vi "TellSelf.vi"(10 "Message":T1 {"MessageMetadata"."AbsoluteTime" format="%<%x %.3X>T"}, 11 "Actor":refnum<class "Actor.lvclass">) -> (0 "Error":errorcluster, 3 "Actor":refnum<class "Actor.lvclass">)   [LabVIEW 2020, in "_Template.lvlib" / "Templates.lvlib" / "{{Name}}Message.lvlib"]
uses:
  {{Name}}Message.lvlib
  {{Name}}Message/{{Name}}Message.lvclass
  C:/jettl-harness/repos/jettl/src/jettl Tools/_Template/Templates/{{Name}}Message/{{Name}}Message/{{Name}}Message.lvclass
  C:/jettl-harness/repos/jettl/src/jettl/jettl/Message/Message.lvclass
  jettl/jettl/jettl.lvlib
  jettl/jettl/Actor/Actor.lvclass
  jettl/jettl/ActorRelation.ctl
  jettl/jettl/ActorLifetime.ctl
  jettl/jettl/MessageMetadata.ctl
  Message.ctl
panel:
  # "This front panel should not be manipulated."
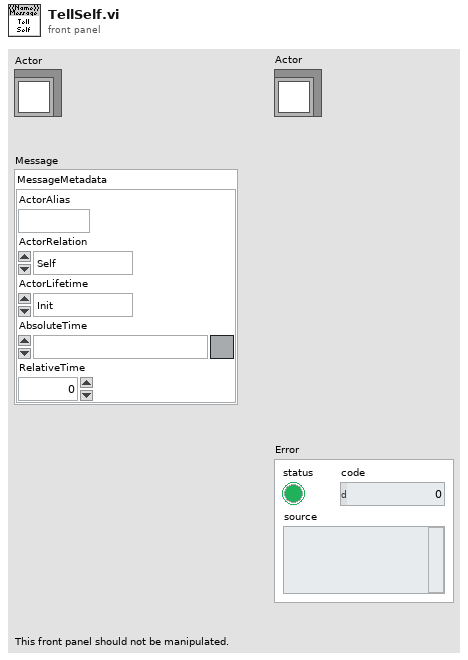
[diagram p1: front panel]
types:
  T1 = typedef "_Template.lvlib/Templates.lvlib/{{Name}}Message.lvlib/Message.ctl" = cluster{"MessageMetadata":T2}
  T2 = typedef "jettl.lvlib/MessageMetadata.ctl" = cluster{"ActorAlias":string, "ActorRelation":T3, "ActorLifetime":T4, "AbsoluteTime":timestamp, "RelativeTime":dbl}
  T3 = typedef "jettl.lvlib/ActorRelation.ctl" = enum16{"Self", "Actor"}
  T4 = typedef "jettl.lvlib/ActorLifetime.ctl" = enum16{"Init", "Spawn", "Setup", "Teardown Before Running", "Running", "Stop Called", "Stopping With Children", "Stopping Without Children", "Teardown After Running", "Stopped"}
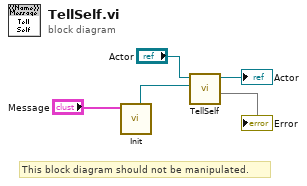
[diagram p0: block diagram]
diagram:
  # "This block diagram should not be manipulated."
  n1 = call "Init.vi"("Message"="Message") -> ("{{Name}}Message"=w5:refnum<class "{{Name}}Message.lvclass">)  [unwired: 10 in]
  n2 = call "TellSelf.vi"("Message"=w5, "Actor"="Actor") -> ("Actor"=→"Actor":refnum<class "Actor.lvclass">, 4:→"Error")  [unwired: 8 in]
